vi "Write Subschedules.vi"(8 "error in (no error)":errorcluster, 10 "Subschedules":refnum<class "Schedule.lvclass">[](array[class]), 11 "Scheduile Array in":refnum<class "Scheduile Array.lvclass">) -> (0 "error out":errorcluster, 3 "Scheduile Array out":refnum<class "Scheduile Array.lvclass">)   [LabVIEW 2015, in "Scheduile Array.lvclass"]
uses:
  Scheduile Array.lvclass
  Schedule.lvclass
  Scheduile Array.lvclass/Scheduile Array.ctl
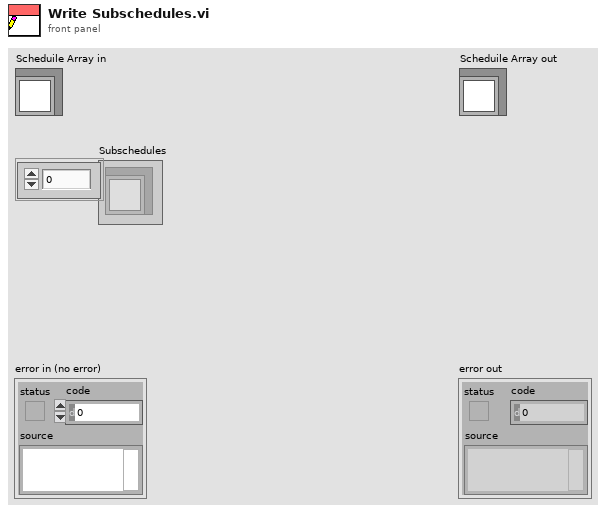
[diagram p1: front panel]
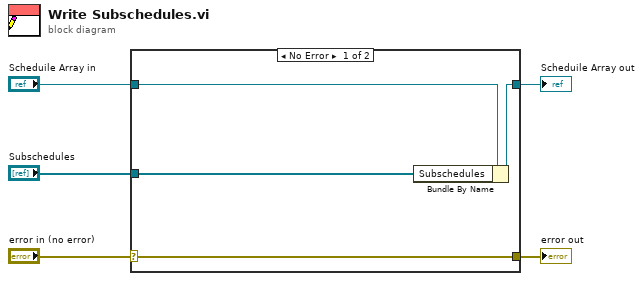
[diagram p0: block diagram]
diagram:
  n1 = case shown="No Error" "error in (no error)" {
    selector: "error in (no error)" -> [w9 w10]
    tunnel: [w9 w10] -> w4
    tunnel: [w7 w11] -> w2
    tunnel: "Scheduile Array in" -> [w8 w11]
    tunnel: "Subschedules" -> [w6 _]
    frame No Error {
      n2 = Bundle By Name(cluster=w8, "Subschedules"=w6) -> (w7:refnum<class "Scheduile Array.lvclass">)
    }
    frame Error {
    }
  }
  "error out" <- w4
  "Scheduile Array out" <- w2
